vi "Get Board Image.vi"(8 "error in (no error)":errorcluster, 10 "Board":string, 11 "RP2040Platform in":refnum<class "RP2040Platform.lvclass">) -> (0 "error out":errorcluster, 2 "Board Image":picture, 3 "RP2040Platform out":refnum<class "RP2040Platform.lvclass">)   [LabVIEW 2020, in "RP2040.lvlib" / "RP2040Platform.lvclass"]
uses:
  RP2040Platform.lvclass
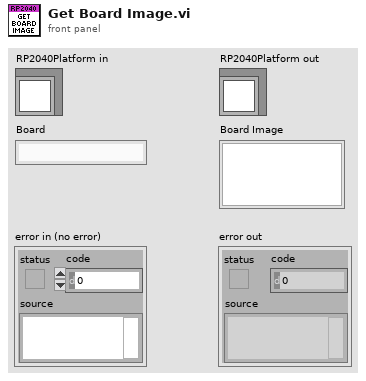
[diagram p1: front panel]
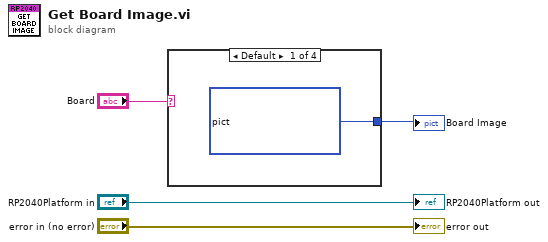
[diagram p0: block diagram]
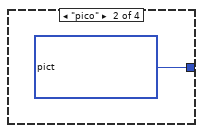
[diagram p2: hidden frame]
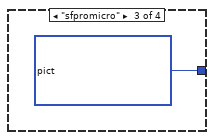
[diagram p3: hidden frame]
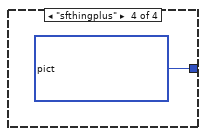
[diagram p4: hidden frame]
diagram:
  n1 = case shown="Default" "Board" {
    tunnel: [picture bytes[22590] ("Board Image") picture bytes[22590] ("new picture") picture bytes[22590] ("new picture") picture bytes[22590] ("new picture")] -> w1
    frame Default {
    }
    frame "pico" {
    }
    frame "sfpromicro" {
    }
    frame "sfthingplus" {
    }
  }
  "Board Image" <- w1
  "error out" <- "error in (no error)"
  "RP2040Platform out" <- "RP2040Platform in"
